vi "CurrentOutput_flt.vi"(7 "y scaled":dbl, 9 "array":dbl[][](array[numeric]), 10 "Z Input":dbl, 11 "X Input":dbl) -> (0 "O":i32, 1 "FW":i32, 2 "FH":i32, 3 "Current Out (pA)":dbl, 4 "Zread":dbl)   [LabVIEW 2019]
uses:
  <vilib>/ptbypt/NI_PtbyPt.lvlib
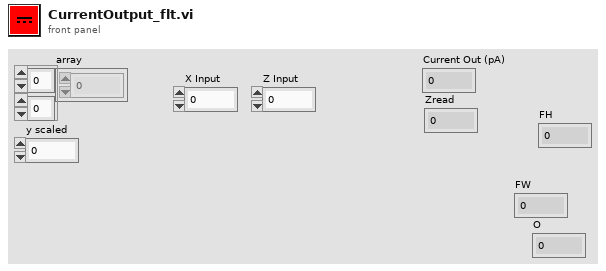
[diagram p1: front panel]
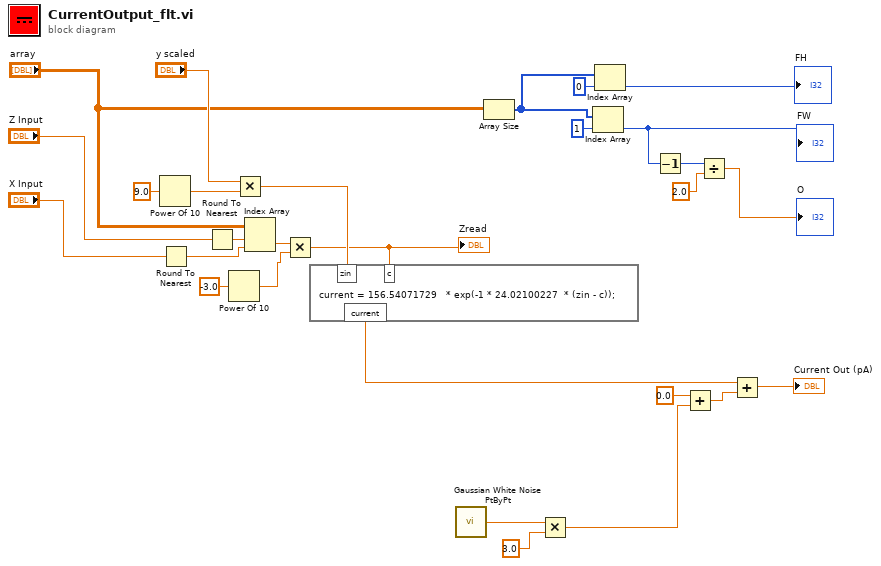
[diagram p0: block diagram]
diagram:
  n1 = Power Of 10(x=9.0) -> (10^x=w27:dbl)
  n2 = Round To Nearest(number="X Input") -> (nearest integer value=w21:dbl)
  n3 = Round To Nearest(number="Z Input") -> (nearest integer value=w28:dbl)
  n4 = Power Of 10(x=-3.0) -> (10^x=w23:dbl)
  n5 = Multiply(x="y scaled", y=w27) -> (x*y=w25:dbl)
  n6 = Index Array(array="array", index (row)=w28, index (col)=w21) -> (element=w18:dbl)
  n7 = Multiply(x=w18, y=w23) -> (x*y=w22:dbl)
  "Zread" <- w22
  n8 = formula code="current = 156.54071729   * exp(-1 * 24.02100227  * (zin - c));"("zin"=w25, "c"=w22) -> ("current"=w10:dbl)
  n9 = call <vilib>:"Gaussian White Noise PtByPt.vi"() -> ("Gaussian white noise"=w16:dbl)  [unwired: 3 in]
  n10 = Array Size(array="array") -> (size(s)=w8:i32[])
  n11 = Multiply(x=w16, y=3.0) -> (x*y=w13:dbl)
  n12 = Index Array(array=w8, index=1) -> (element=w1:i32)
  "FW" <- w1
  n13 = Index Array(array=w8, index=0) -> (element=→"FH":i32)
  n14 = Decrement(x=w1) -> (x-1=w4:i32)
  n15 = Add(x=0.0, y=w13) -> (x+y=w14:dbl)
  n16 = Divide(x=w4, y=2.0) -> (x/y=→"O":dbl)
  n17 = Add(x=w10, y=w14) -> (x+y=→"Current Out (pA)":dbl)
